vi "Getposition.vi"(8 "error in":errorcluster) -> (0 "error out":errorcluster, 3 "Position[µm]":dbl)   [LabVIEW 2017]
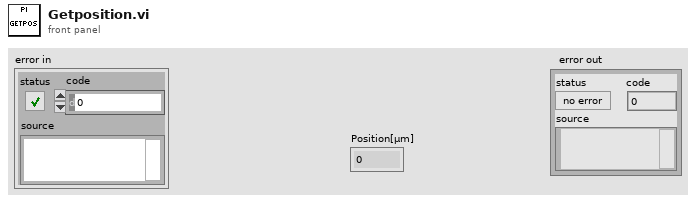
[diagram p1: front panel]
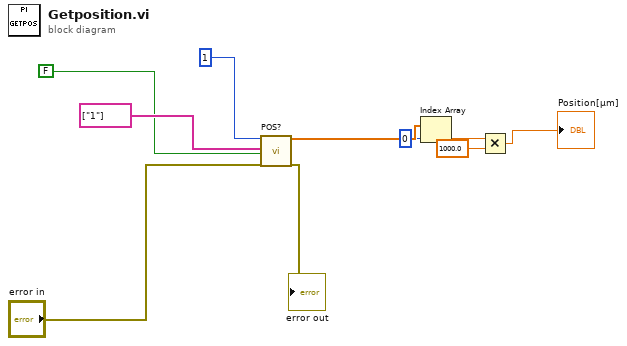
[diagram p0: block diagram]
diagram:
  n1 = call "POS?.vi"("System no."=1, "Axes to query"=string[] ["1"], "All axes?"=FALSE, "error in"="error in") -> ("Position"=w5:dbl[], "error out"=→"error out":errorcluster)  [unwired: 1 in, 13 out]
  n2 = Index Array(array=w5, index=0) -> (element=w3:dbl)
  n3 = Multiply(x=w3, y=1000.0) -> (x*y=→"Position[µm]":dbl)
